vi "TW Resolve Missing Dependency - Custom gRPC Service Core.vi"(8 "error in":errorcluster, 10 "Project Name":string, 11 "Map - LibRef":map{string, refnum<vi>}(c390)) -> (0 "error out":errorcluster)   [LabVIEW 2021, in "Plugin Generator.lvlib"]
uses:
  Plugin Generator.lvlib
panel:
  out "Array":string[](array[string])
  in  "Project Path":path
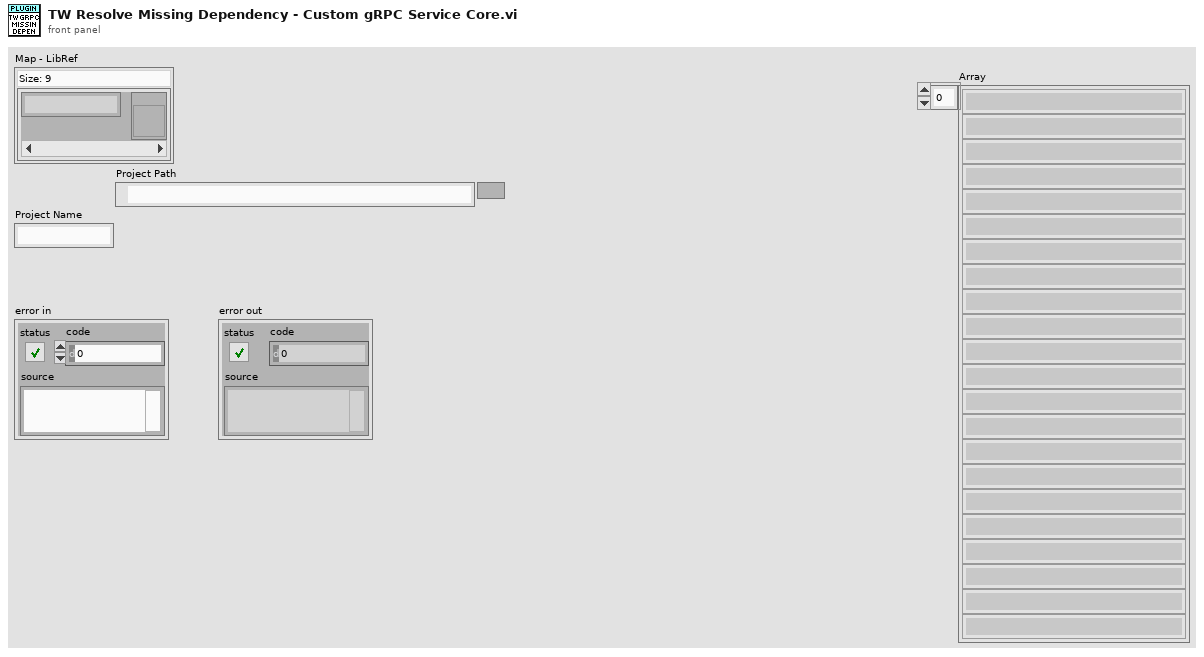
[diagram p1: front panel]
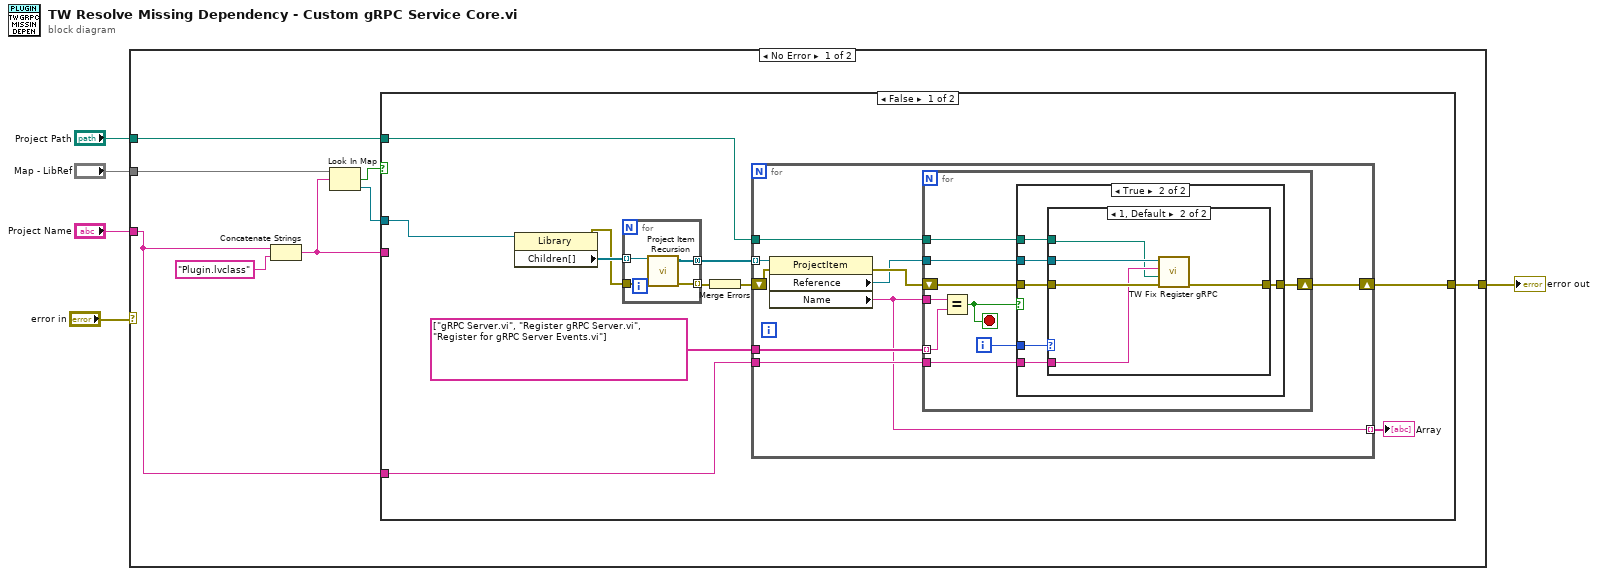
[diagram p0: block diagram]
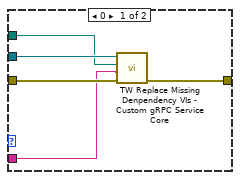
[diagram p3: hidden frame]
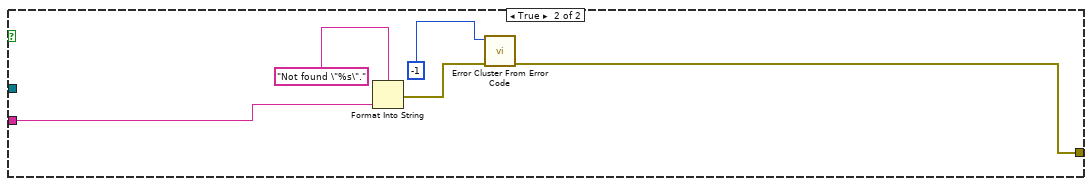
[diagram p4: hidden frame]
diagram:
  n1 = case shown="No Error" "error in" {
    selector: "error in" -> [_ w69]
    tunnel: [w13 w69] -> w5
    tunnel: "Map - LibRef" -> [w9 _]
    tunnel: "Project Name" -> [w7 _]
    tunnel: "Project Path" -> [w6 _]
    frame No Error {
      n2 = Concatenate Strings(w7, "Plugin.lvclass" ("String")) -> (w8:string)
      n3 = Look In Map(map=w9, key=w8) -> (key not found?=w11:bool, value=w12:refnum<vi>)  [unwired: 1 in]
      n4 = case shown="False" w11 {
        tunnel: w12 -> [w24 _]
        tunnel: [w16 w65] -> w13
        tunnel: w7 -> [w17 _]
        tunnel: w8 -> [_ w64]
        tunnel: w6 -> [w15 _]
        frame False {
          n5 = property class="Library"(reference=w24) -> (error out=w22:errorcluster, "Children[]"=w23:refnum<vi>[])  [unwired: 1 in, 1 out]
          n6 = for {
            tunnel: w23 -> [w63] mode=indexing
            tunnel: [w62] -> w21 mode=concatenating
            tunnel: w22 -> [w61]
            tunnel: [w60] -> w19 mode=indexing
            n7 = call "Project Item Recursion.vi"("error in"=w61, "TargetItem in"=w63) -> ("error out"=w60:errorcluster, "TargetItem out"=w62:refnum<vi>[])  [unwired: 8 in]
          }
          n8 = Merge Errors(w19) -> (w20:errorcluster)
          n9 = for {
            tunnel: w21 -> [w33] mode=indexing
            tunnel: string[] ["gRPC Server.vi", "Register gRPC Server.vi", "Register for gRPC Server Events.vi"] -> [w32]
            tunnel: w15 -> [w28]
            tunnel: w17 -> [w27]
            shift-right: [w26] -> w16
            shift-left: w20 -> [w31]
            tunnel: [w25] -> w14 mode=indexing
            n10 = property class="ProjectItem"(reference=w33, error in=w31) -> (error out=w30:errorcluster, "Reference"=w29:refnum<vi>, "Name"=w25:string)  [unwired: 1 out]
            n11 = for {
              tunnel: w32 -> [w42] mode=indexing
              tunnel: w25 -> [w41]
              tunnel: w29 -> [w39]
              tunnel: w28 -> [w36]
              tunnel: w27 -> [w35]
              shift-right: [w34] -> w26
              shift-left: w30 -> [w40]
              i -> [w37]
              stop <- w38 stop-if-true
              n12 = Equal?(x=w41, y=w42) -> (x = y?=w38:bool)
              n13 = case shown="True" w38 {
                tunnel: w40 -> [w43 w48]
                tunnel: w39 -> [_ w49]
                tunnel: w37 -> [_ w47]
                tunnel: w36 -> [_ w46]
                tunnel: w35 -> [_ w45]
                tunnel: [w43 w44] -> w34
                frame False {
                }
                frame True {
                  n14 = case shown="1, Default" w47 {
                    tunnel: w49 -> [w54 w58]
                    tunnel: w48 -> [w53 w59]
                    tunnel: w46 -> [w52 w56]
                    tunnel: w45 -> [w51 w57]
                    tunnel: [w50 w55] -> w44
                    frame 0 {
                      n15 = call "TW Replace Missing Denpendency VIs - Custom gRPC Service Core.vi"("error in"=w53, "gRPC Service Name"=w51, "Project Path"=w52, "VI Refnum"=w54) -> ("error out"=w50:errorcluster)  [unwired: 7 in]
                    }
                    frame 1, Default {
                      n16 = call "TW Fix Register gRPC.vi"("error in"=w59, "Project Path"=w56, "gRPC Service Name"=w57, "VI Refnum"=w58) -> ("error out"=w55:errorcluster)  [unwired: 7 in]
                    }
                  }
                }
              }
            }
          }
          "Array" <- w14
        }
        frame True {
          n17 = Format Into String(format string="Not found \"%s\"." ("error message (\"\")"), w64) -> (error out=w67:errorcluster)  [unwired: 2 in, 1 out]
          n18 = call <vilib>:"Error Cluster From Error Code.vi"("error in (no error)"=w67, "error code (0)"=-1) -> ("error out"=w65:errorcluster)  [unwired: 7 in]
        }
      }
    }
    frame Error {
    }
  }
  "error out" <- w5
